vi "Set Distance Matrix.vi"(0 "GMaps API in":refnum<class "GMaps API.lvclass">, 1 "Path":T1={"Color"="", "Weight"="", "Destination State"="", "Destination City"=" ", "Destination Street"="", "Origin State"="", "Origin City"=" ", "Origin Street"=""}, 5 "error in (no error)":errorcluster) -> (14 "GMaps API out":refnum<class "GMaps API.lvclass">, 19 "error out":errorcluster)   [LabVIEW 2016, in "GMaps API.lvclass"]
doc: "Sets Distance Matrix based on the recommended route between start and end points."
uses:
  GMaps API.lvclass
  Controls/Path.ctl
  GMaps API.lvclass/GMaps API.ctl
  <vilib>/regexp/Match Regular Expression.xnode
  <vilib>/httpClient/LabVIEWHTTPClient.lvlib
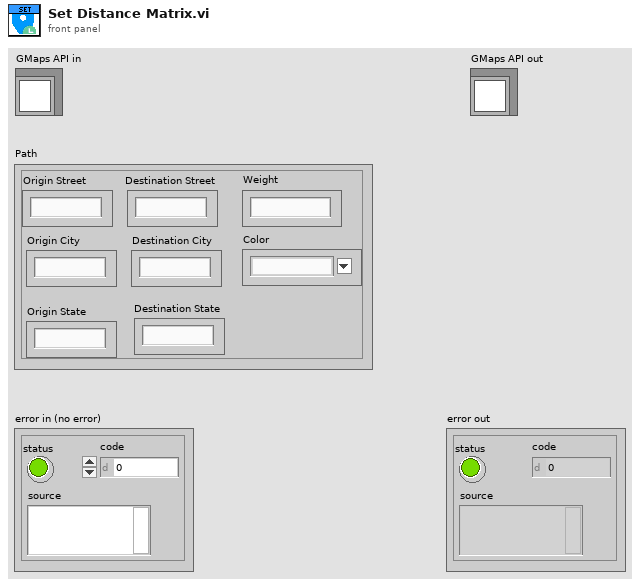
[diagram p1: front panel]
types:
  T1 = typedef "GMaps API.lvclass/Path.ctl" = cluster{"Color":string, "Weight":string, "Destination State":string, "Destination City":string, "Destination Street":string, "Origin State":string, "Origin City":string, "Origin Street":string}
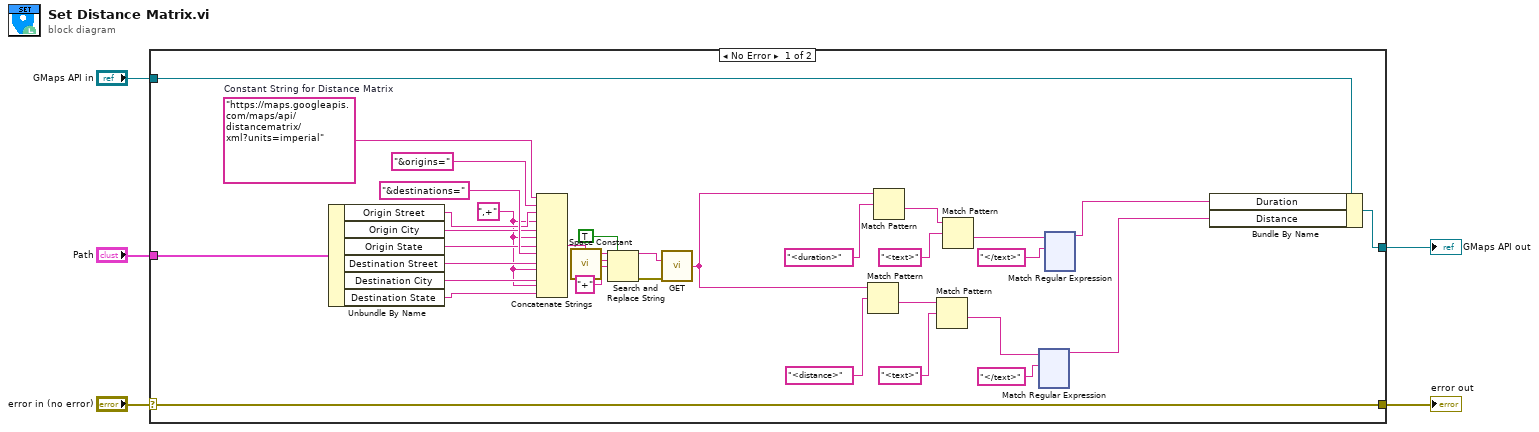
[diagram p0: block diagram]
diagram:
  n1 = case shown="No Error" "error in (no error)" {
    selector: "error in (no error)" -> [w38 w268]
    tunnel: [w38 w268] -> w4
    tunnel: [w36 w267] -> w2
    tunnel: "GMaps API in" -> [w37 w267]
    tunnel: "Path" -> [w13 _]
    frame No Error {
      w6 = ",+" ("string")
      w18 = "https://maps.googleapis.com/maps/api/distancematrix/xml?units=imperial"  # Constant String for Distance Matrix
      n2 = Unbundle By Name(w13) -> ("Origin Street"=w12:string, "Origin City"=w11:string, "Origin State"=w10:string, "Destination Street"=w9:string, "Destination City"=w8:string, "Destination State"=w7:string)
      n3 = Concatenate Strings(w18, "&origins=" ("string"), w12, w6, w11, w6, w10, "&destinations=" ("string"), w9, w6, w8, w6, w7) -> (w30:string)
      n4 = call <vilib>:"Space Constant.vi"() -> ("String"=w31:string)
      n5 = Search and Replace String(replace all?=TRUE ("replace all? (F)"), input string=w30, search string=w31, replace string="+" ("replace string (\"\")")) -> (result string=w34:string, error out=w33:errorcluster)  [unwired: 4 in, 2 out]
      n6 = call <vilib>:"GET.vi"("url"=w34, "error in (no error)"=w33) -> ("body"=w22:string)  [unwired: 10 in, 3 out]
      n7 = Match Pattern(string=w22, regular expression="<distance>") -> (after substring=w25:string)  [unwired: 4 out]
      n8 = Match Pattern(string=w22, regular expression="<duration>") -> (after substring=w23:string)  [unwired: 4 out]
      n9 = Match Pattern(string=w25, regular expression="<text>" ("Directly Before Latitude info")) -> (after substring=w19:string)  [unwired: 4 out]
      n10 = Match Pattern(string=w23, regular expression="<text>" ("Directly After Latitude info")) -> (after substring=w20:string)  [unwired: 4 out]
      n11 = xnode "Match Regular Expression"("input string"=w19, "regular expression"="</text>" ("Directly After Latitude info")) -> ("before match"=w14:string)  [unwired: 4 in, 4 out]
      n12 = xnode "Match Regular Expression"("input string"=w20, "regular expression"="</text>") -> ("before match"=w15:string)  [unwired: 4 in, 4 out]
      n13 = Bundle By Name(cluster=w37, "Duration"=w15, "Distance"=w14) -> (w36:refnum<class "GMaps API.lvclass">)
    }
    frame Error {
    }
  }
  "error out" <- w4
  "GMaps API out" <- w2
